vi "s(i).vi"(1 "s":i32, 2 "r":dbl, 3 "m":i32, 4 "n":i32) -> (0 "R Sumand nm (r)":dbl)   [LabVIEW 2020, in "Zernike Polynome.lvlib"]
doc: "Calculation of the Sumand i."
uses:
  Zernike Polynome.lvlib
  <vilib>/gmath/NI_Gmath.lvlib
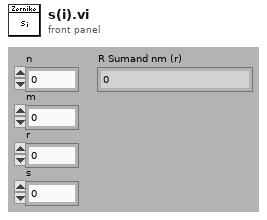
[diagram p1: front panel]
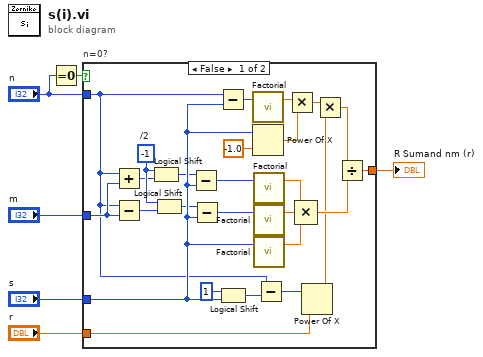
[diagram p0: block diagram]
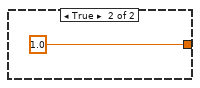
[diagram p2: hidden frame]
diagram:
  n1 = Equal To 0?(x="n") -> (x = 0?=w2:bool)
  n2 = case "n=0?" shown="False" w2 {
    tunnel: "s" -> [w28 _]
    tunnel: "n" -> [w7 _]
    tunnel: "m" -> [w12 _]
    tunnel: [w11 1.0] -> w4
    tunnel: "r" -> [w10 _]
    frame False {
      w23 = -1  # /2
      n3 = Add(x=w7, y=w12) -> (x+y=w21:i32)
      n4 = Subtract(x=w7, y=w12) -> (x-y=w22:i32)
      n5 = Logical Shift(y=w23, x=w21) -> (x << y=w24:i32)
      n6 = Logical Shift(y=w23, x=w22) -> (x << y=w25:i32)
      n7 = Subtract(x=w24, y=w28) -> (x-y=w26:i32)
      n8 = Subtract(x=w25, y=w28) -> (x-y=w27:i32)
      n9 = Subtract(x=w7, y=w28) -> (x-y=w15:i32)
      n10 = Logical Shift(y=1, x=w28) -> (x << y=w9:i32)
      n11 = call <vilib>:"Factorial.vi"("n"=w15) -> ("n!"=w14:dbl)  [unwired: 2 in]
      n12 = Power Of X(1:-1.0 ("x"), 2:w28) -> (0:w17:dbl)
      n13 = call <vilib>:"Factorial.vi"("n"=w26) -> ("n!"=w29:dbl)  [unwired: 2 in]
      n14 = call <vilib>:"Factorial.vi"("n"=w27) -> ("n!"=w30:dbl)  [unwired: 2 in]
      n15 = call <vilib>:"Factorial.vi"("n"=w28) -> ("n!"=w31:dbl)  [unwired: 2 in]
      n16 = Subtract(x=w7, y=w9) -> (x-y=w8:i32)
      n17 = Multiply(x=w14, y=w17) -> (x*y=w18:dbl)
      n18 = Compound Arithmetic op=MULTIPLY(w29, w30, w31) -> (w32:dbl)
      n19 = Power Of X(1:w10, 2:w8) -> (0:w19:dbl)
      n20 = Multiply(x=w18, y=w19) -> (x*y=w20:dbl)
      n21 = Divide(x=w20, y=w32) -> (x/y=w11:dbl)
    }
    frame True {
    }
  }
  "R Sumand nm (r)" <- w4
